vi "Set Data Value.vi"(8 "error in (no error)":errorcluster, 9 "Data":dbl, 10 "Some flag":bool, 11 "numericPayload in":refnum<class "numericPayload.lvclass">) -> (0 "error out":errorcluster, 3 "numericPayload out":refnum<class "numericPayload.lvclass">)   [LabVIEW 2017, in "messagesPayload.lvlib" / "numericPayload.lvclass"]
uses:
  numericPayload.lvclass
  numericPayload.lvclass/numericPayload.ctl
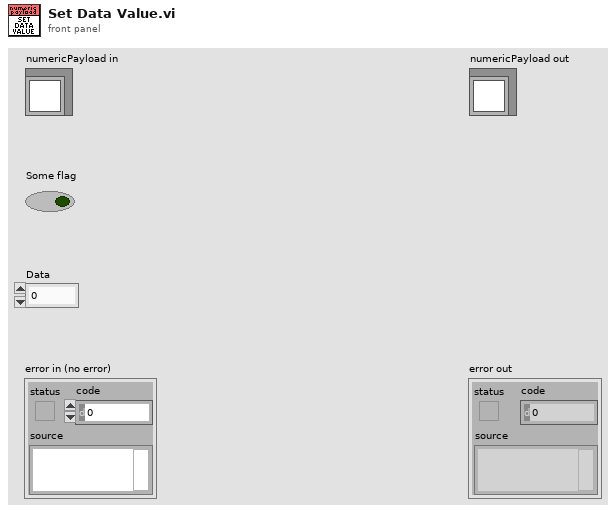
[diagram p1: front panel]
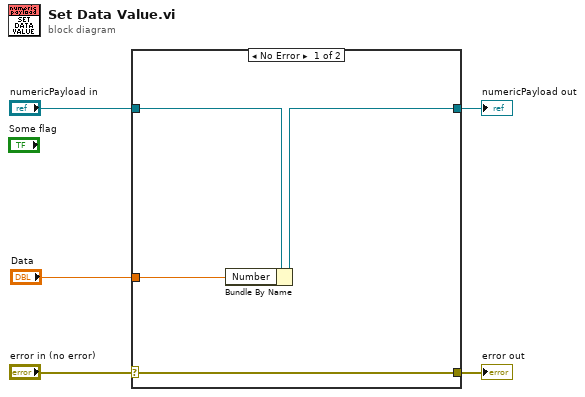
[diagram p0: block diagram]
diagram:
  n1 = case shown="No Error" "error in (no error)" {
    selector: "error in (no error)" -> [w8 w11]
    tunnel: [w8 w11] -> w4
    tunnel: [w7 w10] -> w2
    tunnel: "numericPayload in" -> [w9 w10]
    tunnel: "Data" -> [w6 _]
    frame No Error {
      n2 = Bundle By Name(cluster=w9, "Number"=w6) -> (w7:refnum<class "numericPayload.lvclass">)
    }
    frame Error {
    }
  }
  "error out" <- w4
  "numericPayload out" <- w2
